vi "Write T.vi"(8 "error in (no error)":errorcluster, 10 "T":dbl, 11 "ePAS Cell Data in":refnum<class "ePAS Cell Data.lvclass">) -> (0 "error out":errorcluster, 3 "ePAS Cell Data out":refnum<class "ePAS Cell Data.lvclass">)   [LabVIEW 2014, in "ePAS Library.lvlib" / "ePAS Cell Data.lvclass"]
uses:
  ePAS Cell Data.lvclass
  ePAS Cell Data.lvclass/ePAS Cell Data.ctl
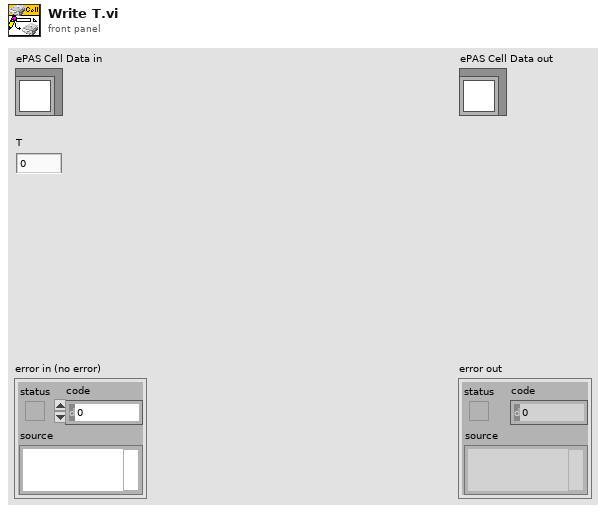
[diagram p1: front panel]
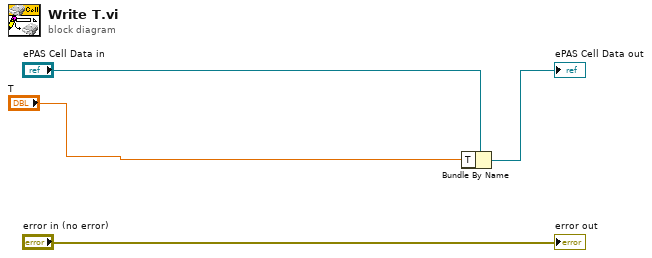
[diagram p0: block diagram]
diagram:
  n1 = Bundle By Name(cluster="ePAS Cell Data in", "T"="T") -> (→"ePAS Cell Data out":refnum<class "ePAS Cell Data.lvclass">)
  "error out" <- "error in (no error)"
